vi "Read Travel Units.vi"(8 "error in (no error)":errorcluster, 11 "Force Test Stand in":refnum<class "Force Test Stand.lvclass">) -> (0 "error out":errorcluster, 2 "Travel Units":T1, 3 "Force Test Stand out":refnum<class "Force Test Stand.lvclass">)   [LabVIEW 2018, in "Force Test Stand.lvlib" / "Force Test Stand.lvclass"]
uses:
  Force Test Stand.lvclass
  Custom Controls/Travel Units.ctl
  Force Test Stand.lvclass/Force Test Stand.ctl
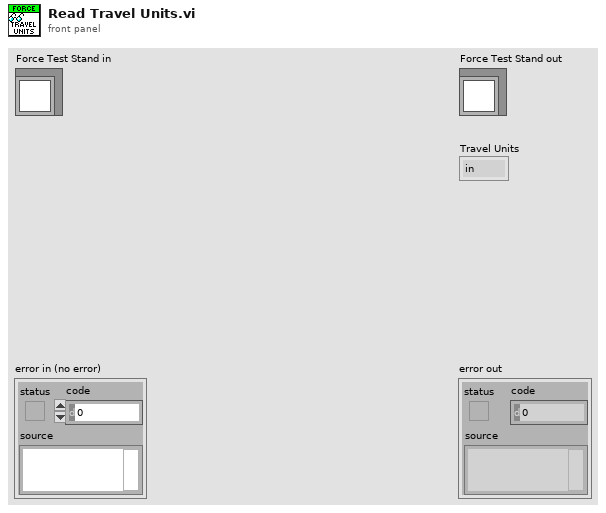
[diagram p1: front panel]
types:
  T1 = typedef "Force Test Stand.lvlib/Force Test Stand.lvclass/Travel Units.ctl" = enum16{"in", "mm"}
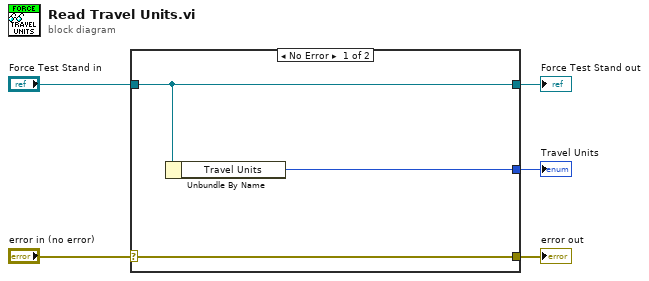
[diagram p0: block diagram]
diagram:
  n1 = case shown="No Error" "error in (no error)" {
    selector: "error in (no error)" -> [w8 w9]
    tunnel: [w8 w9] -> w4
    tunnel: [w7 w10] -> w2
    tunnel: "Force Test Stand in" -> [w7 w10]
    tunnel: [w6 _] -> w1
    frame No Error {
      n2 = Unbundle By Name(w7) -> ("Travel Units"=w6:T1)
    }
    frame Error {
    }
  }
  "error out" <- w4
  "Force Test Stand out" <- w2
  "Travel Units" <- w1
